vi "set_config_cluster.vi"(8 "error in (no error)":errorcluster, 10 "config cluster variant":variant, 11 "TrajectoryRK110916Throughput in":refnum<class "TrajectoryRK110916Throughput.lvclass">) -> (0 "error out":errorcluster, 3 "TrajectoryRK110916Throughput out":refnum<class "TrajectoryRK110916Throughput.lvclass">)   [LabVIEW 2010, in "TrajectoryRK110916Throughput.lvclass"]
uses:
  TrajectoryRK110916Throughput.lvclass
  TrajectoryRK110916Throughput.lvclass/TrajectoryRK110916Throughput.ctl
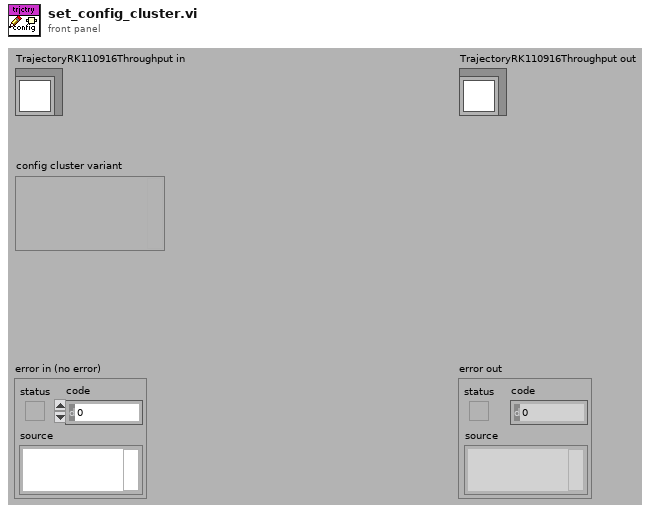
[diagram p1: front panel]
types:
  T1 = typedef "TrajectoryRK110916Throughput.lvclass/config_data_cluster.ctl" = cluster{"FGPA clockspeed":dbl}
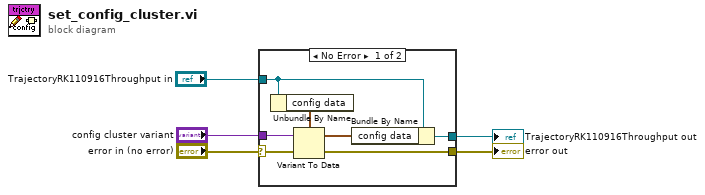
[diagram p0: block diagram]
diagram:
  n1 = case shown="No Error" "error in (no error)" {
    selector: "error in (no error)" -> [w12 w14]
    tunnel: [w11 w14] -> w4
    tunnel: [w6 w13] -> w2
    tunnel: "TrajectoryRK110916Throughput in" -> [w10 w13]
    tunnel: "config cluster variant" -> [w8 _]
    frame No Error {
      n2 = Unbundle By Name(w10) -> ("config data"=w7:T1)
      n3 = Variant To Data(error in=w12, Variant=w8, type=w7) -> (error out=w11:errorcluster, data=w9:T1)
      n4 = Bundle By Name(cluster=w10, "config data"=w9) -> (w6:refnum<class "TrajectoryRK110916Throughput.lvclass">)
    }
    frame Error {
    }
  }
  "error out" <- w4
  "TrajectoryRK110916Throughput out" <- w2
